vi "timing-on-host.vi"() -> ()   [LabVIEW 2020]
uses:
  <vilib>/Utility/file.llb/Write Delimited Spreadsheet (I64).vi
panel:
  in  "timing data out":path
  out "x-y":u32
  out "delta t min":dbl
  out "delta t max":dbl
  out "iterations":i32
  out "timing array":i32[](array[numeric])
  in  "stop":bool
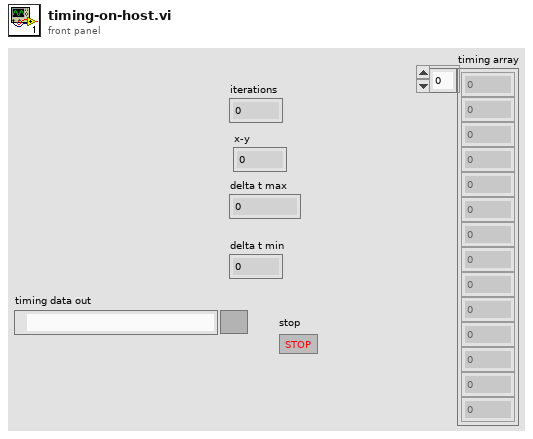
[diagram p1: front panel]
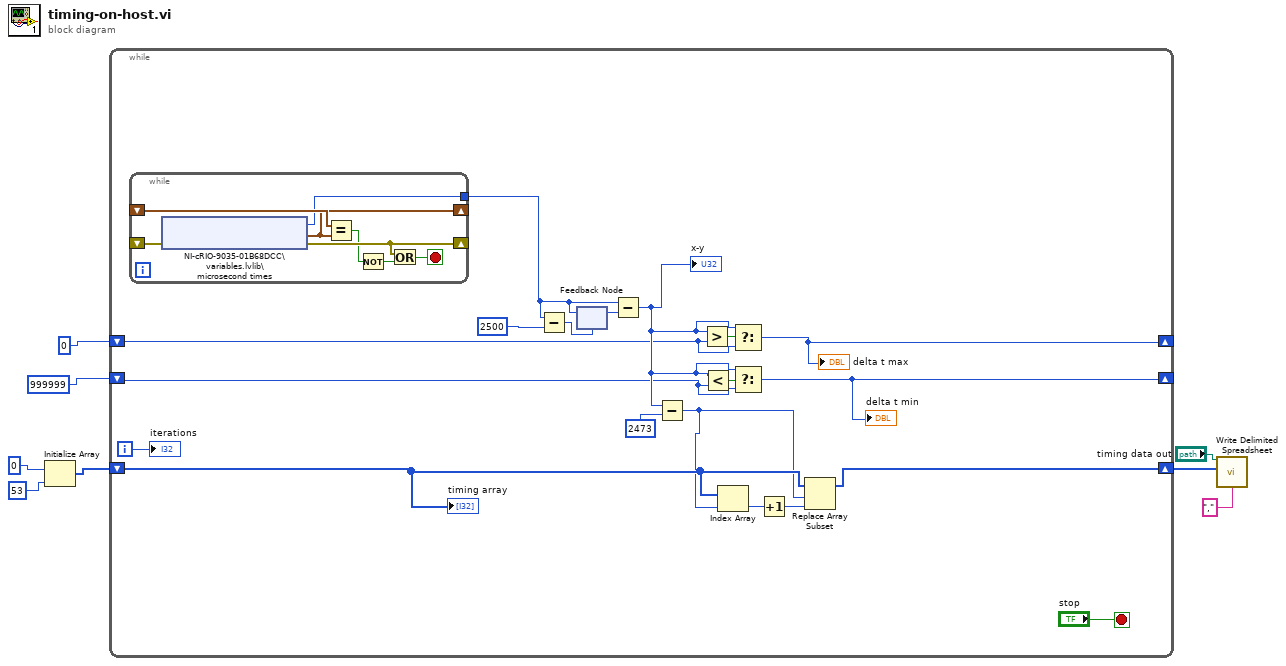
[diagram p0: block diagram]
diagram:
  n1 = Initialize Array(0, 53) -> (w4:i32[])
  n2 = while {
    shift-right: [w20] -> _
    shift-left: 0 -> [w22]
    shift-right: [w19] -> _
    shift-left: 999999 -> [w21]
    shift-right: [w11] -> w3
    shift-left: w4 -> [w12]
    i -> [w18]
    stop <- "stop" stop-if-true
    n3 = while {
      shift-right: [w28] -> _
      shift-left: _ -> [w34]
      shift-right: [w33] -> _
      shift-left: _ -> [w35]
      tunnel: [w30] -> w17
      stop <- w29 stop-if-true
      n4 = shared-variable "NI-cRIO-9035-01B68DCC\\variables.lvlib\\microsecond times"(error in=w35) -> (w30:i32, error out=w33:errorcluster, w28:timestamp)
      n5 = Equal?(x=w34, y=w28) -> (x = y?=w31:bool)
      n6 = Not(x=w31) -> (.not. x?=w32:bool)
      n7 = Or(x=w33, y=w32) -> (x .or. y?=w29:bool)
    }
    n8 = Subtract(x=w17, y=2500) -> (x-y=w16:i32)
    n9 = feedback #1(w16) -> (w27:i32)
    n10 = feedback-in #1(w17) -> ()
    n11 = Subtract(x=w17, y=w27) -> (x-y=w24:i32)
    "x-y" <- w24
    n12 = Subtract(x=w24, y=2473) -> (x-y=w10:i32)
    n13 = Greater?(x=w24, y=w22) -> (0:w26:bool)
    n14 = Less?(x=w24, y=w21) -> (x < y?=w25:bool)
    n15 = Index Array(array=w12, index=w10) -> (element=w13:i32)
    n16 = Select(t=w24, s=w26, f=w22) -> (s? t:f=w20:i32)
    "delta t max" <- w20
    n17 = Select(t=w24, s=w25, f=w21) -> (s? t:f=w19:i32)
    "delta t min" <- w19
    n18 = Increment(x=w13) -> (x+1=w14:i32)
    n19 = Replace Array Subset(array=w12, new element=w14, index=w10) -> (w11:i32[])
    "iterations" <- w18
    "timing array" <- w12
  }
  n20 = call-poly <vilib>:"Write Delimited Spreadsheet.vi"("file path (dialog if empty)"="timing data out", "1D data"=w3, "delimiter (\\t)"=",") -> ()  [unwired: 11 in, 2 out]
